vi "Main.vi"(8 "error in (no error)":errorcluster) -> (0 "error out":errorcluster)   [LabVIEW 2020, in "main.lvlib"]
uses:
  main.lvlib
  report format.ctl
  Module Data--cluster.ctl
  core/core_data/completed_tour.ctl
  core/core_data/chessboard_index.ctl
  core/core_data/tour type (enum).ctl
  core/core_data/chess_square--chess notation.ctl
  core/core_data/file--enum.ctl
  core/core_data/rank--enum.ctl
  config_buttons--enum.ctl
  update_completed_tour_text_indicator arguments.ctl
  create completed tour report (minimal).vi
  create completed tour report (detailed).vi
  <vilib>/Utility/error.llb/Clear Errors.vi
  core/core_wait (global variable).vi
  core/pause after every move (global variable).vi
  core/pause (global variable).vi
  convert--tour to string (minimal format).vi
  convert--tour to string (chessboard format).vi
  PTRL/string/Number (DBL) to comma delimited string.vi
  PTRL/dev_and_debug_tools/dev_and_debug_tools.lvlib
  PTRL/errors/errors.lvlib
  PTRL/GUI_tools/GUI_tools.lvlib
  queues/queue_core_loop/queue_core_loop.lvlib
  queues/queue_display_loop_1/queue_display_loop_1.lvlib
  global_stop_flag/global_stop_flag.lvlib
  app_data/app_data.lvlib
  status_text_indicator/Status_Text_Indicator.lvlib
  core/core.lvlib
  core/core_data/core_data.lvlib
  PTRL/timing_utilities/timing_utilities.lvlib
  app_log/app_log.lvlib
  PTRL/pro_dev_tools/pro_dev_tools.lvlib
  PTRL/string/string.lvlib
  stopwatch_timer/stopwatch_timer.lvlib
panel:
  out "avg. tour finding speed":string
  out "no. of completed tours":u64
  in  "Report format":T1
  in  "Log reports to file?":bool=TRUE caption="Log completed tour reports to file?"
  in  "open log in Sublime Text":bool
  in  "open log in Notepad":bool
  in  "open log folder":bool
  out "log file path":string caption="Log file path"
  out "avg. move speed":string
  out "no. of moves forward and backward in the last second":string
  out "total no. of moves":string
  out "total no. of moves backward":string
  out "total no. of moves forward":string
  in  "pause after every move?":bool caption="Pause after every move"
  in  "no. of ms to wait after each move":u32 max=5000 format="%d ms"
  out "no. of complete tours":string caption="no. of completed tours"
  out "complete_tour currently displayed":u64 caption="completed_tour currently displayed"
  in  "display_latest":bool=TRUE caption="Always show the latest completed tour"
  in  "display_previous":bool
  in  "display_next":bool
  out "complete_tour":string caption="Completed tour reports"
  out "running time":string
  out "total no. of moves":u64
  out "chessboard":bool[][](array[boolean]) caption="Chessboard"
  out "display loop 2":i32
  out "The tour":string caption="The current knight's tour"
  in  "Status":string
  in  "stop":bool
  in  "pause":bool
  in  "start":bool
  out "display loop 1":i32
  out "core loop":i32
  out "error case":errorcluster
  in  "top_left":u32(colorbox)=13434847
  in  "bottom_right":u32(colorbox)=16764108
  out "No. of states":i32
  out "MHL state transition (index 0 = oldest)":string[](array[string])
  out "MHL iteration":i32
  out "EHL iteration":i32
  out "Pre-loop init":errorcluster
  in  "Insert Unrecognised MHL command":bool
  in  "Insert error EHL":bool
  in  "Insert error MHL":bool
  # "Visible to user"
  # "Knight Tour"
  # "Tutorial section"
  # "Use the controls below to slow down the execution and/or to pause after every knight move."
  # "Invisible to user"
  # "8"
  # "7"
  # "6"
  # "5"
  # "4"
  # "3"
  # "2"
  # "1"
  # "a"
  # "b"
  # "c"
  # "d"
  # "e"
  # "f"
  # "g"
  # "h"
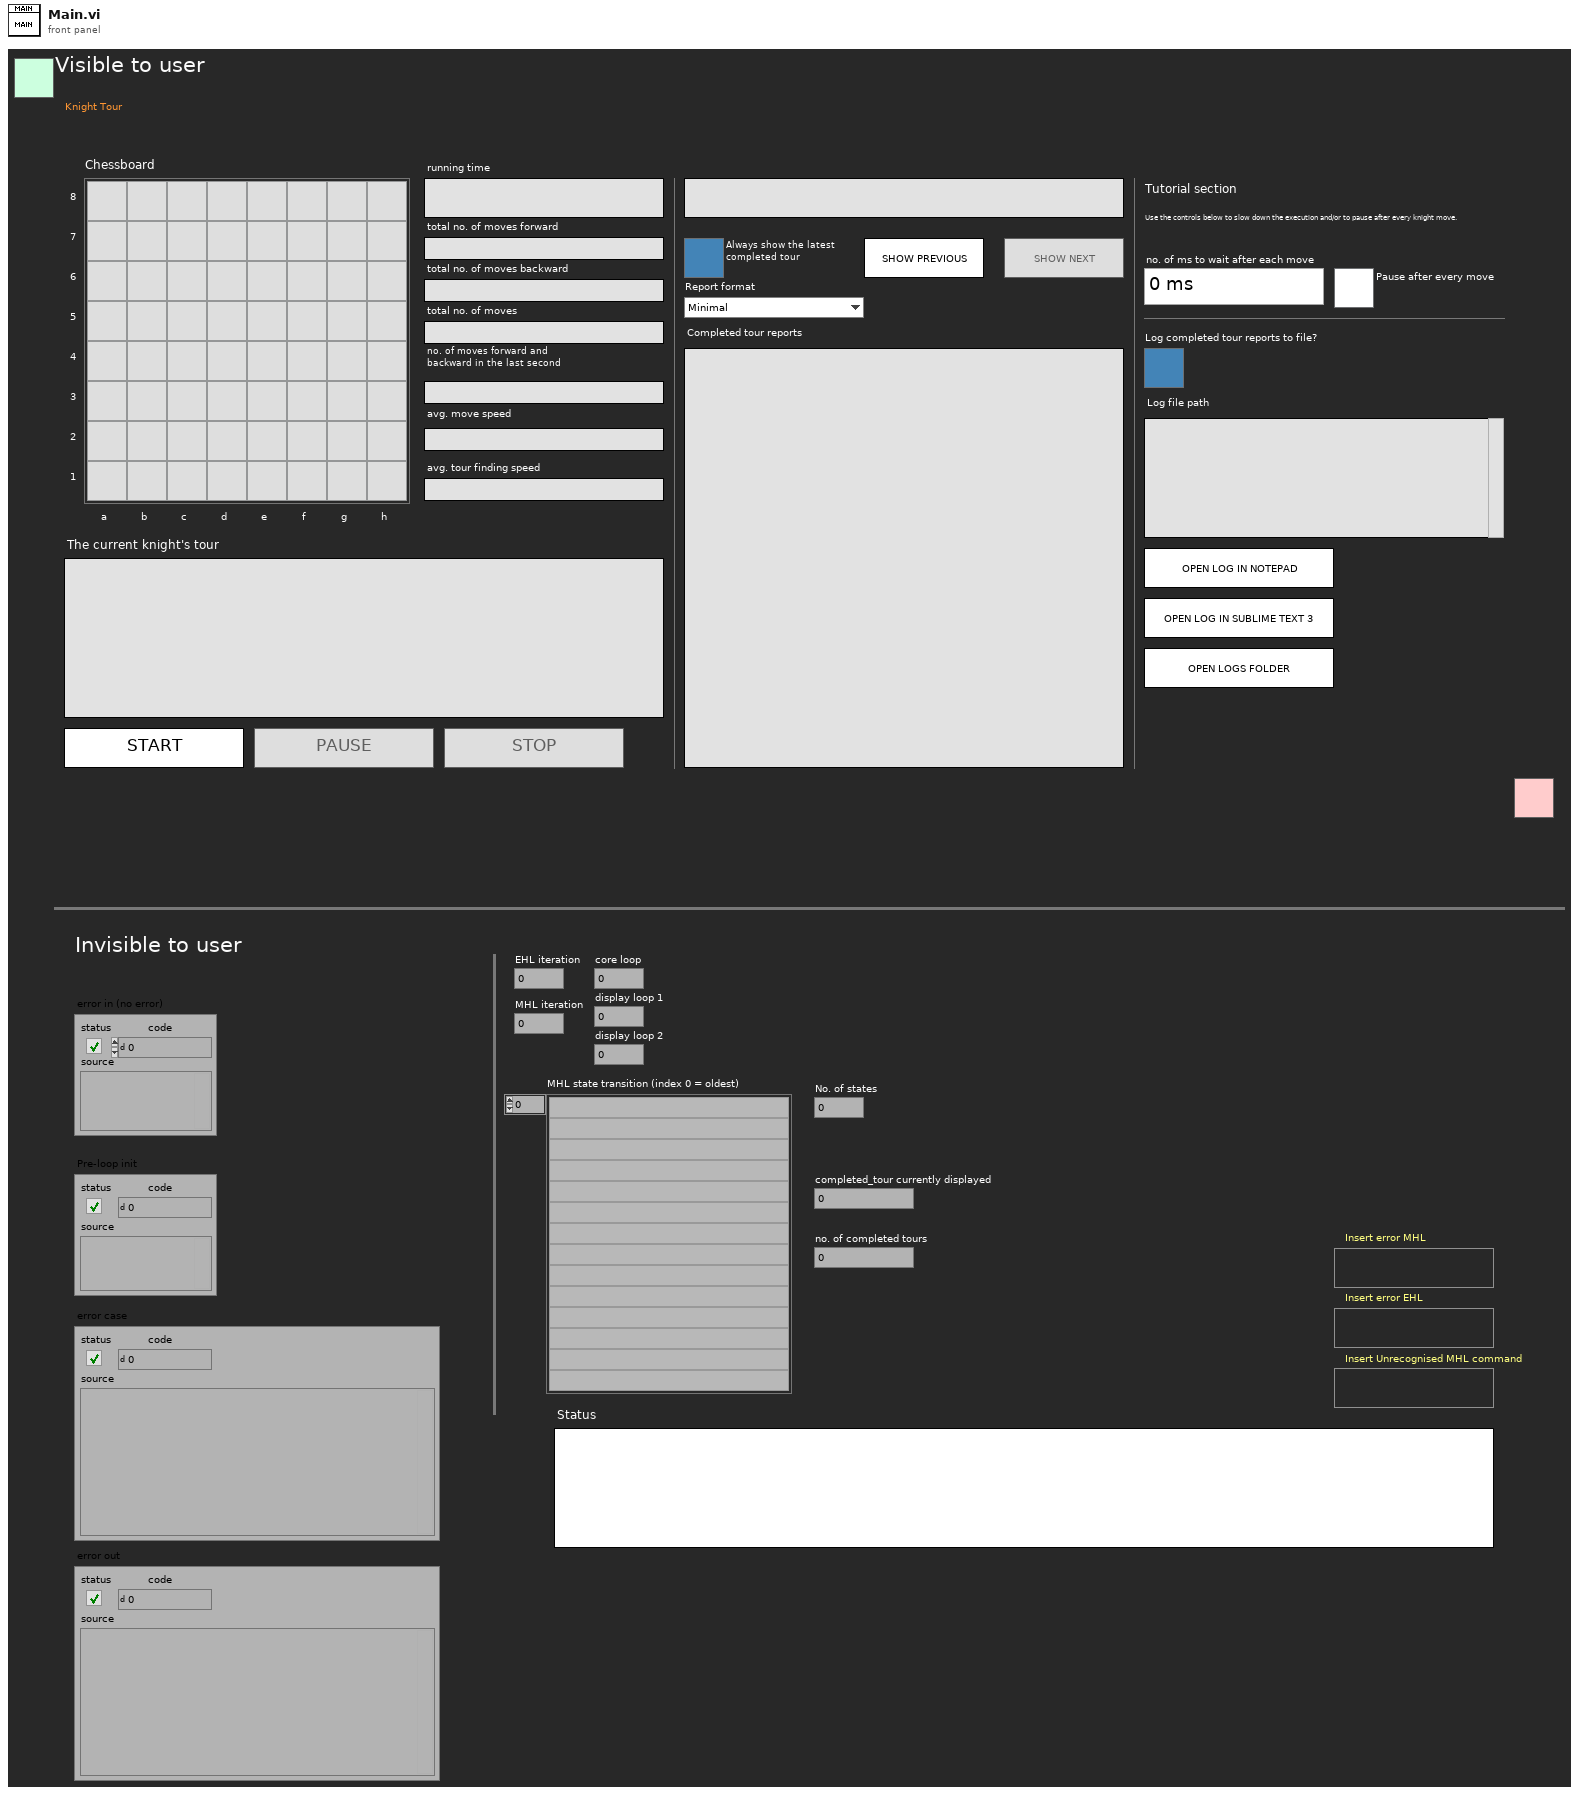
[diagram p1: front panel]
types:
  T1 = typedef "main.lvlib/report format.ctl" = enum16{"Minimal", "Detailed"}
  T2 = enum8{"Enabled", "Disabled", "Disabled and Grayed Out"}
  T3 = typedef "main.lvlib/Module Data--cluster.ctl" = cluster{"complete_tours":T4[], "no. of complete tours":u64, "complete_tour currently displayed":u64}
  T4 = typedef "core.lvlib/core_data.lvlib/completed_tour.ctl" = cluster{"complete_tour":T5[], "start square":string, "end square":string, "tour type":T6, "start_time":timestamp, "end_time":timestamp, "duration (seconds)":dbl, "duration (formatted string)":string, "no. of moves forward":u64, "no. of moves backward":u64, "total no. of moves since core started running":u64}
  T5 = typedef "core.lvlib/core_data.lvlib/chessboard_index.ctl" = cluster{"row":u8, "column":u8}
  T6 = typedef "core.lvlib/core_data.lvlib/tour type (enum).ctl" = enum16{"open", "closed"}
  T7 = typedef "main.lvlib/config_buttons--enum.ctl" = enum16{"tour_not_running", "tour_running", "tour_paused"}
  T8 = typedef "main.lvlib/update_completed_tour_text_indicator arguments.ctl" = cluster{"Completed tour paragraph":string, "tour number":u64}
  T9 = typedef "core.lvlib/core_data.lvlib/chess_square--chess notation.ctl" = cluster{"file":T10, "rank":T11}
  T10 = typedef "core.lvlib/core_data.lvlib/file--enum.ctl" = enum16{"a", "b", "c", "d", "e", "f", "g", "h"}
  T11 = typedef "core.lvlib/core_data.lvlib/rank--enum.ctl" = enum16{"1", "2", "3", "4", "5", "6", "7", "8"}
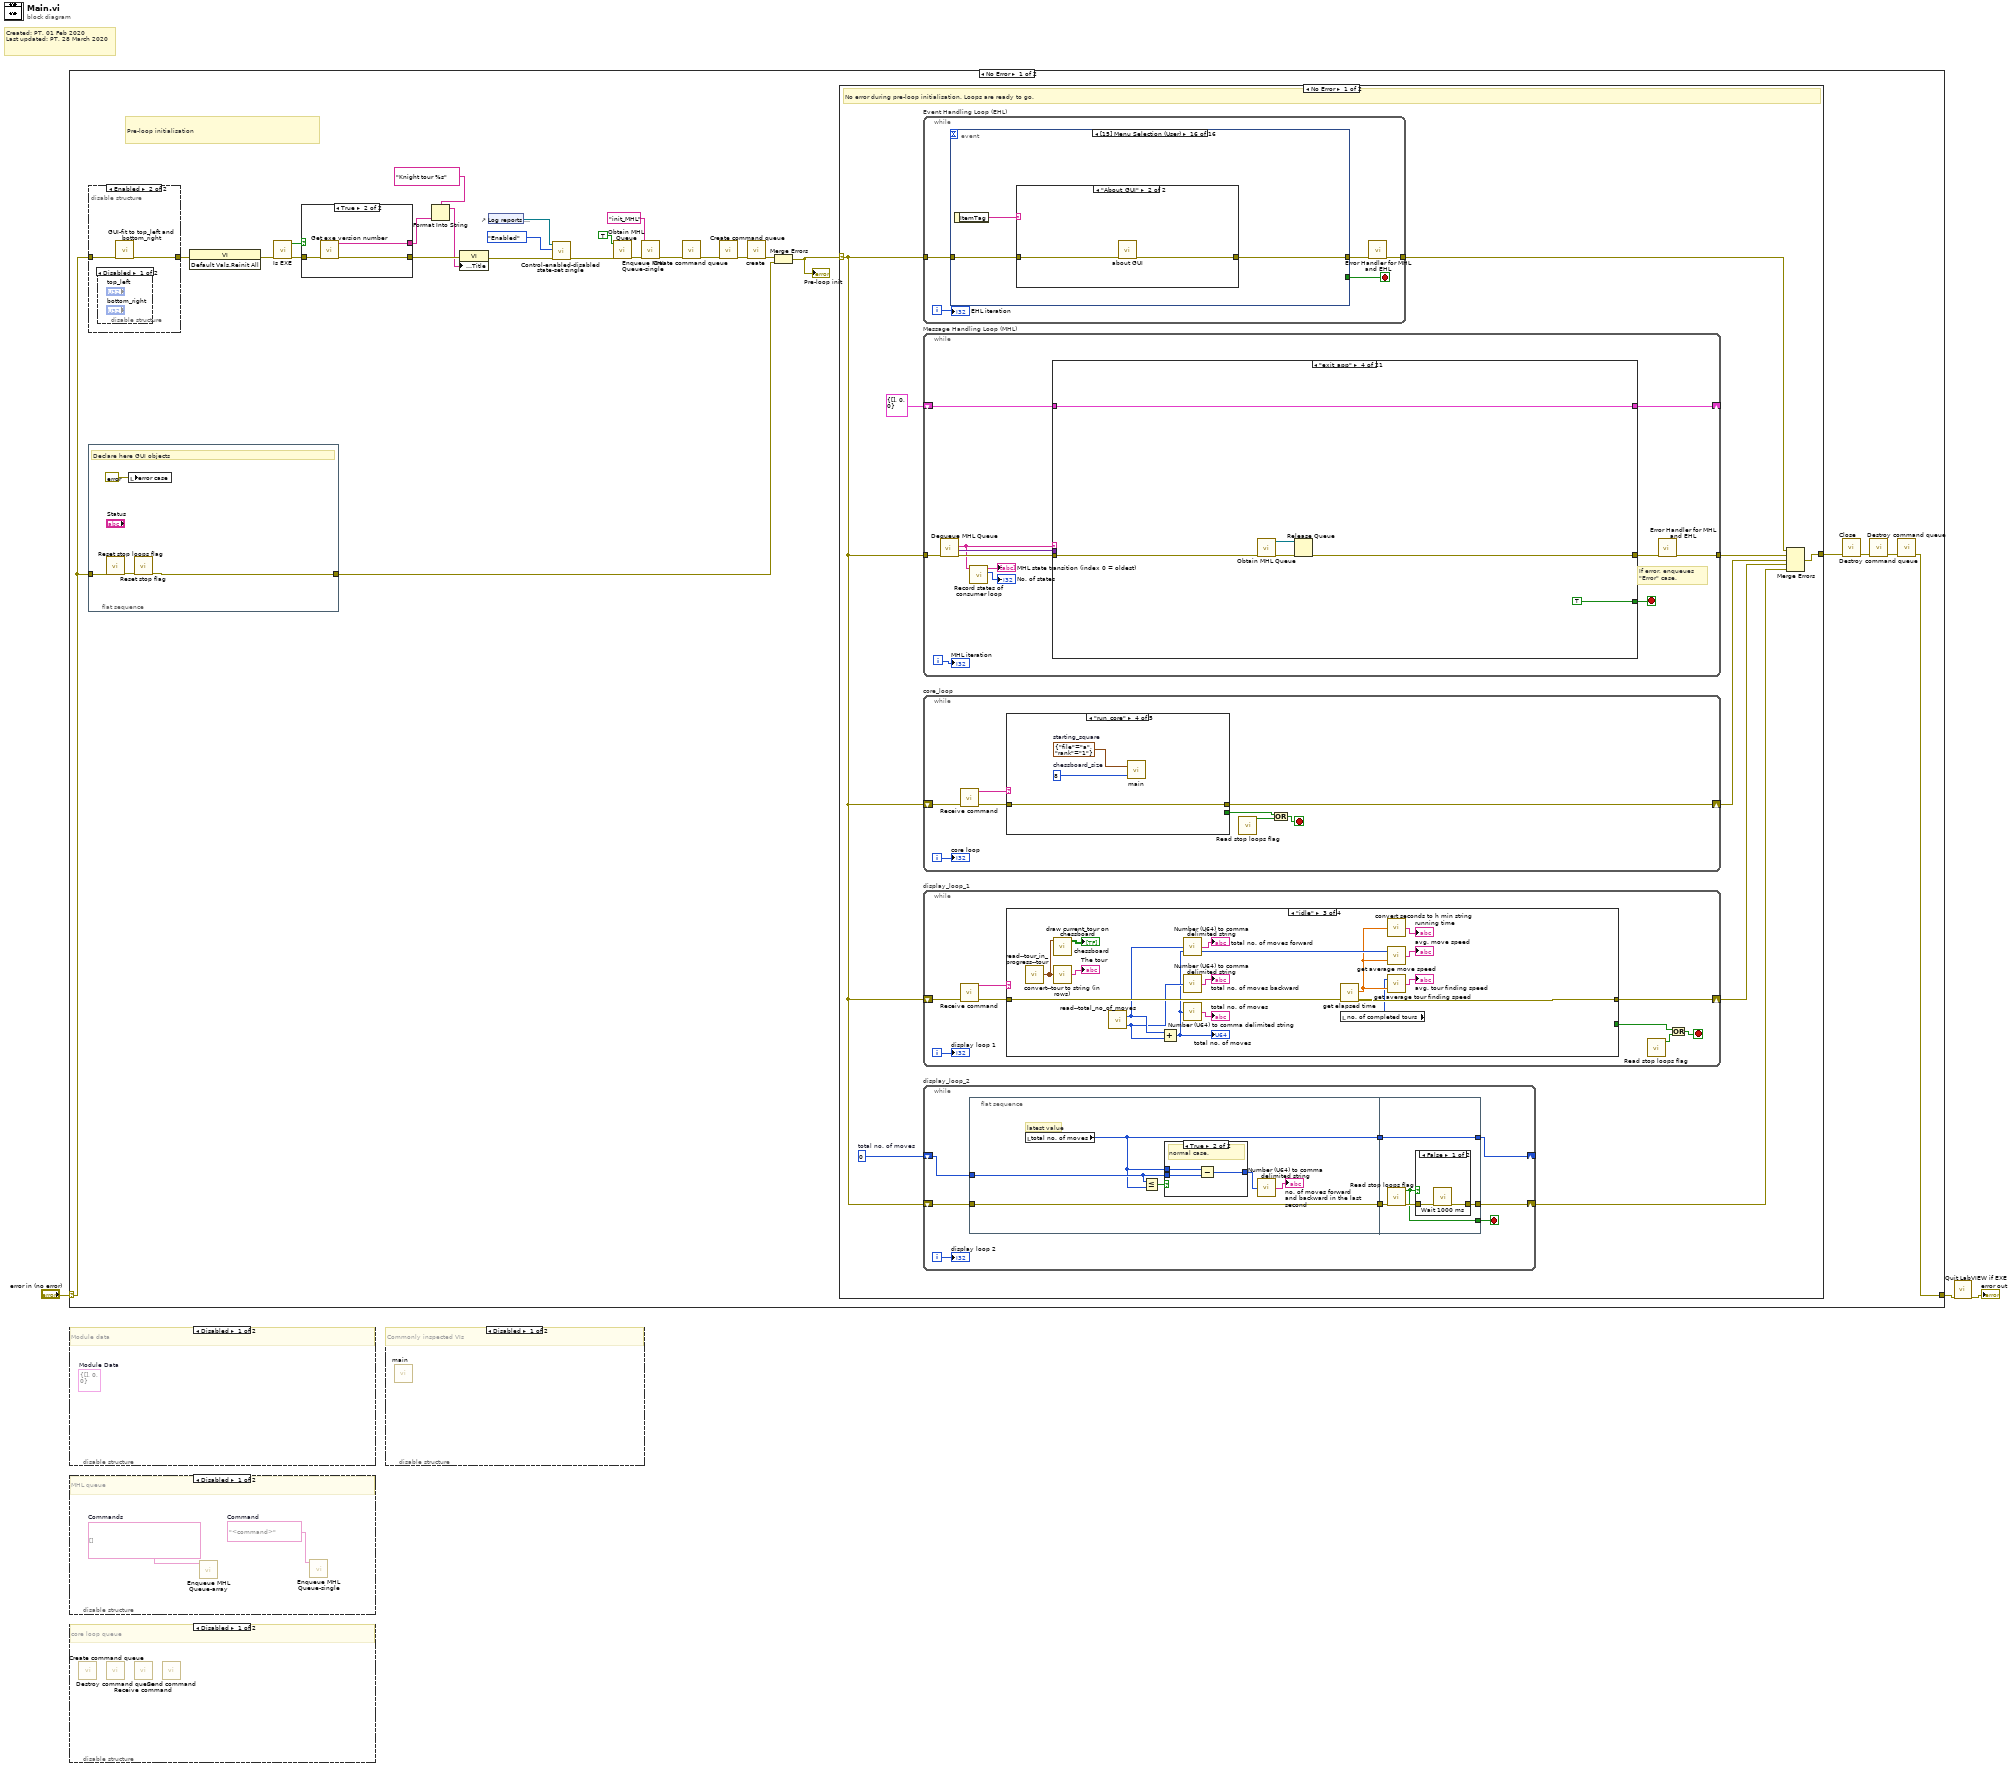
[diagram p0: block diagram]
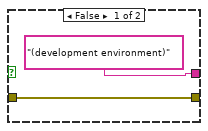
[diagram p2: hidden frame]
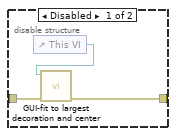
[diagram p3: hidden frame]
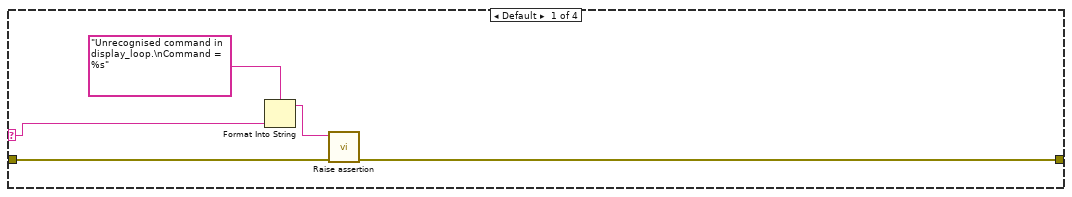
[diagram p5: hidden frame]
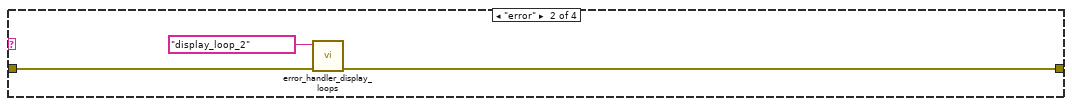
[diagram p6: hidden frame]
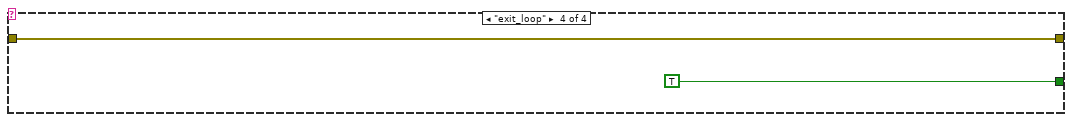
[diagram p7: hidden frame]
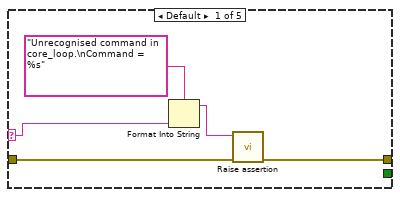
[diagram p8: hidden frame]
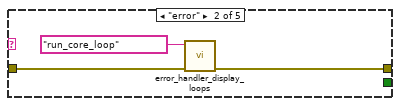
[diagram p9: hidden frame]
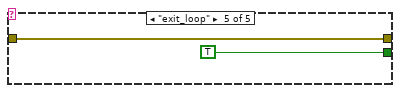
[diagram p11: hidden frame]
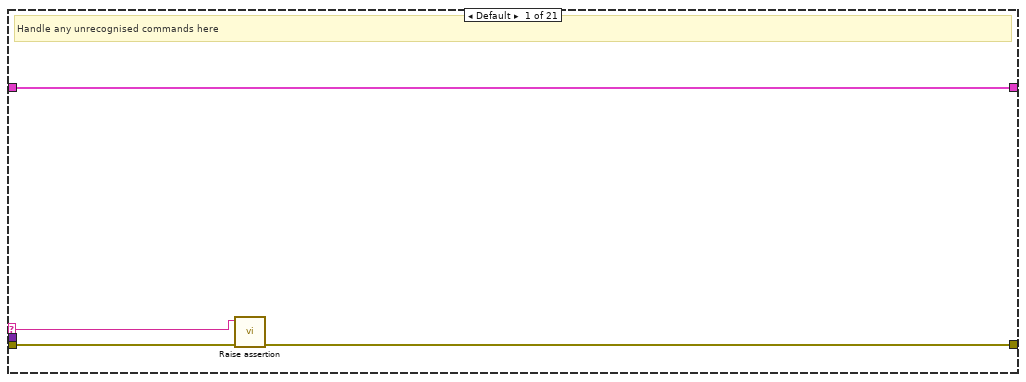
[diagram p12: hidden frame]
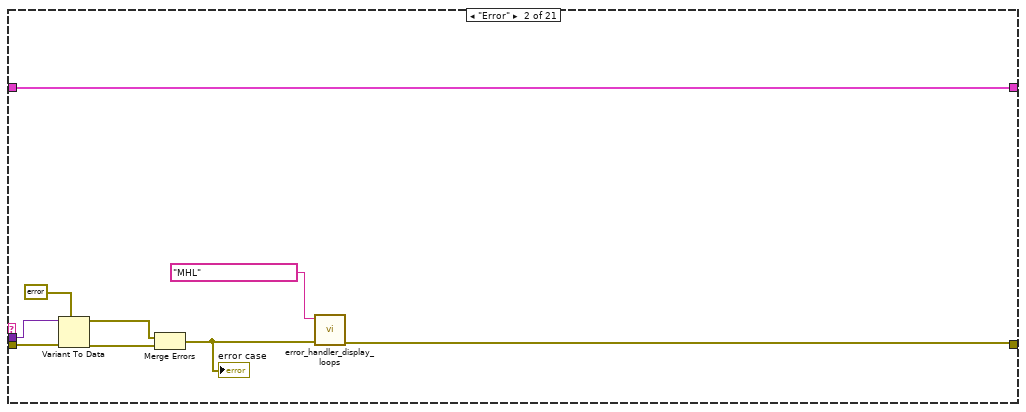
[diagram p13: hidden frame]
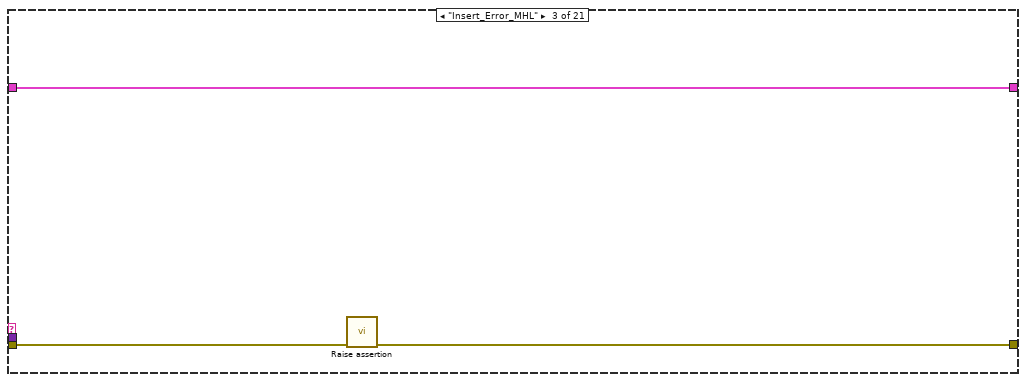
[diagram p14: hidden frame]
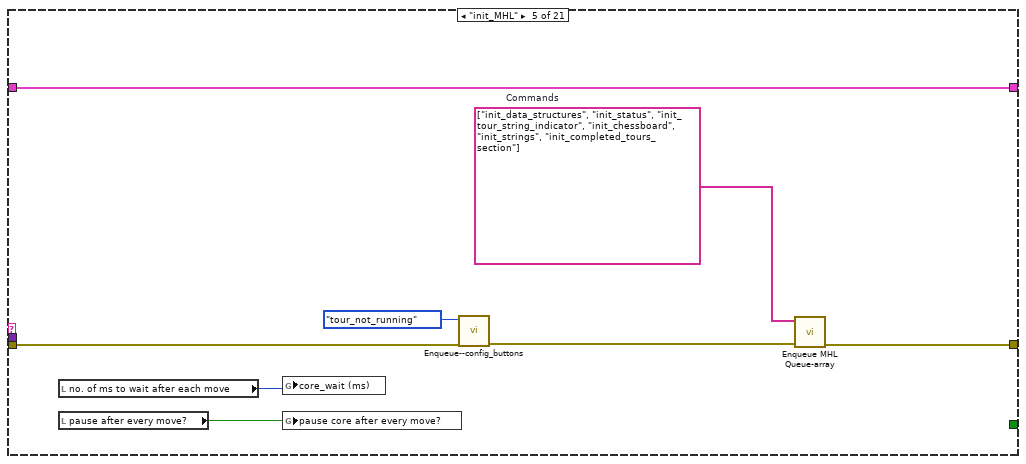
[diagram p15: hidden frame]
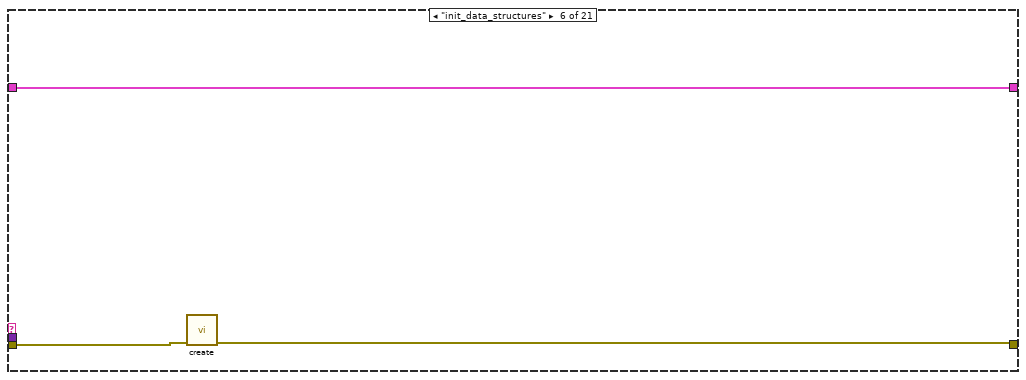
[diagram p16: hidden frame]
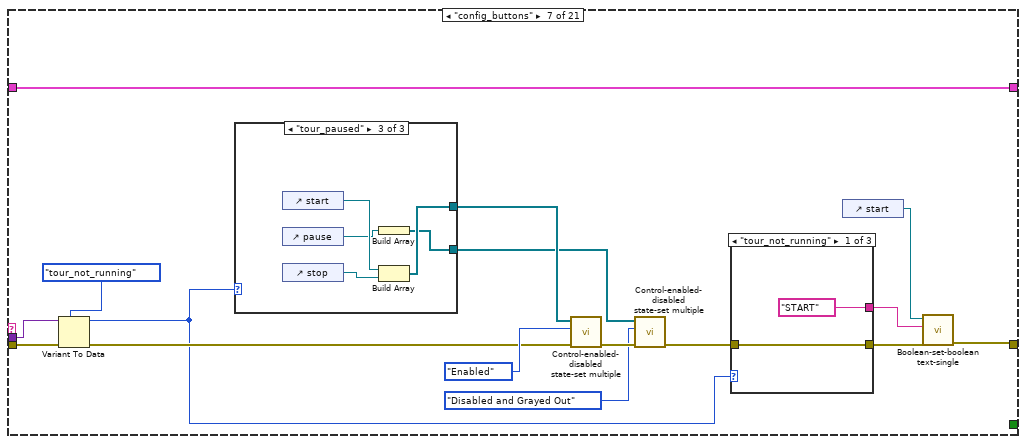
[diagram p17: hidden frame]
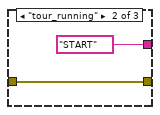
[diagram p18: hidden frame]
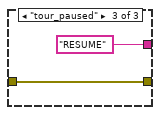
[diagram p19: hidden frame]
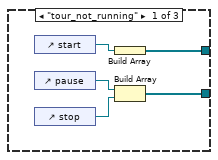
[diagram p20: hidden frame]
diagram:
  # "Created: PT, 01 Feb 2020\nLast updated: PT, 28 March 2020"
  n1 = case shown="No Error" "error in (no error)" {
    selector: "error in (no error)" -> [w24 w530]
    tunnel: [w29 w530] -> w2
    frame No Error {
      # "Pre-loop initialisation"
      n2 = disable-structure shown="Enabled" {
        disable-tunnel: w24 -> [w41 w43]
        disable-tunnel: [w40 w42] -> w27
        frame Disabled {
          n3 = control-ref of="This VI"() -> (w39:refnum<vi>)
          n4 = call "GUI-fit to largest decoration and center.vi"("error in (no error)"=w41, "VI Ref (calling VI)"=w39) -> ("error out"=w40:errorcluster)  [unwired: 9 in]
        }
        frame Enabled {
          n5 = disable-structure shown="Disabled" {
            frame Disabled {
            }
            frame Enabled {
            }
          }
          n6 = call "GUI-fit to top_left and bottom_right.vi"("error in (no error)"=w43) -> ("error out"=w42:errorcluster)  [unwired: 10 in]
        }
      }
      n7 = flat-sequence {
        tunnel: w24 -> [w37]
        tunnel: [w35] -> w22
        frame #0 {
          # "Declare here GUI objects"
          n8 = call "Reset stop loops flag.vi"("error in (no error)"=w37) -> ("error out"=w36:errorcluster)  [unwired: 10 in]
          n9 = local write "error case"(errorcluster {"status"=FALSE, "code"=0, "source"=""} ("error case")) -> ()
          n10 = call "Reset stop flag.vi"("error in (no error)"=w36) -> ("error out"=w35:errorcluster)  [unwired: 10 in]
        }
      }
      n11 = invoke class="VI" method="Default Vals.Reinit All"(error in=w27) -> (error out=w17:errorcluster)  [unwired: 2 in, 2 out]
      n12 = call "Is EXE.vi"("error in (no error)"=w17) -> ("error out"=w15:errorcluster, "T = is EXE"=w13:bool)  [unwired: 8 in, 1 out]
      n13 = case shown="True" w13 {
        tunnel: w15 -> [w31 w34]
        tunnel: [w31 w33] -> w14
        tunnel: ["(development environment)" w32] -> w10
        frame False {
        }
        frame True {
          n14 = call "Get exe version number.vi"("error in"=w34) -> ("error out"=w33:errorcluster, "EXE version number"=w32:string)  [unwired: 9 in]
        }
      }
      n15 = Format Into String(format string="Knight tour %s", w10) -> (resulting string=w11:string)  [unwired: 2 in, 1 out]
      n16 = property class="VI"(error in=w14, "Front Panel Window:Title"=w11) -> (error out=w16:errorcluster)  [unwired: 1 in, 1 out]
      n17 = control-ref of="Log reports to file?"() -> (w8:refnum<vi>)
      n18 = call "Control-enabled-disabled state-set single.vi"("error in (no error)"=w16, "State"=T2."Enabled", "Control ref in"=w8) -> ("error out"=w9:errorcluster)  [unwired: 7 in, 1 out]
      n19 = call "Obtain MHL Queue.vi"("ErrorIn"=w9, "Create New (F)"=TRUE) -> ("ErrorOut"=w28:errorcluster)  [unwired: 8 in, 1 out]
      n20 = call "Enqueue MHL Queue-single.vi"("ErrorIn"=w28, "Command"="init_MHL") -> ("ErrorOut"=w18:errorcluster)  [unwired: 9 in]
      n21 = call "Create command queue.vi"("error in (no error)"=w18) -> ("error out"=w21:errorcluster)  [unwired: 10 in]
      n22 = call "Create command queue.vi"("error in (no error)"=w21) -> ("error out"=w19:errorcluster)  [unwired: 10 in]
      n23 = call "create.vi"("error in"=w19) -> ("error out"=w6:errorcluster)  [unwired: 10 in]
      n24 = Merge Errors(w6, w22) -> (w23:errorcluster)
      "Pre-loop init" <- w23
      n25 = case shown="No Error" w23 {
        selector: w23 -> [w44 w529]
        tunnel: [w51 w529] -> w5
        frame No Error {
          w45 = u64 0  # total no. of moves
          # "No error during pre-loop initialisation. Loops are ready to go."
          n26 = while "Event Handling Loop (EHL)" {
            tunnel: w44 -> [w404]
            tunnel: [w402] -> w52
            i -> [w400]
            stop <- w403 stop-if-true
            n27 = event shown="[15] Menu Selection (User)" {
              selector: _ -> [_ _ _ _ _ _ _ _ _ _ _ _ _ _ _ _]
              dyn-events: _ -> [_ _ _ _ _ _ _ _ _ _ _ _ _ _ _ _]
              timeout: _ -> [_ _ _ _ _ _ _ _ _ _ _ _ _ _ _ _]
              tunnel: w404 -> [w407 w420 w422 w425 w428 w434 w437 w444 w451 w454 w456 w458 w462 w474 w487 w500]
              tunnel: [w405 _ _ _ _ _ _ _ _ _ _ _ _ _ _ _] -> w403
              tunnel: [w409 w421 w423 w426 w432 w435 w441 w443 w450 w453 w456 w458 w463 w473 w486 w499] -> w401
              event Panel Close? {
                n28 = event-data() -> ()  [unwired: 1 in, 1 out]
                n29 = call "dialogue--exit_app.vi"("error in (no error)"=w407) -> ("error out"=w408:errorcluster, "T = exit was pressed"=w406:bool)  [unwired: 9 in]
                n30 = case shown="True" w406 {
                  tunnel: w408 -> [w411 w418]
                  tunnel: [w411 w416] -> w409
                  tunnel: [_ TRUE] -> w405
                  frame False {
                  }
                  frame True {
                    w413 = "exit_loop" ("command")
                    n31 = call "Enqueue--exit_app.vi"("error in (no error)"=w418) -> ("error out"=w415:errorcluster)  [unwired: 10 in]
                    n32 = call "Send command.vi"("error in (no error)"=w415, "command"=w413) -> ("error out"=w414:errorcluster)  [unwired: 9 in]
                    n33 = call "Send command.vi"("error in (no error)"=w414, "command"=w413) -> ("error out"=w412:errorcluster)  [unwired: 9 in]
                    n34 = call "Set stop loops flag.vi"("error in (no error)"=w412) -> ("error out"=w416:errorcluster)  [unwired: 10 in]
                  }
                }
                n35 = event-data("Discard?"=TRUE) -> ()  [unwired: 1 in, 1 out]
              }
              event "Insert error MHL": Value Change {
                # "This case is very useful to simulate the behaviour of the MHL (and of the GUI as a whole), when an error happens in the MHL loop."
                n36 = event-data() -> ()  [unwired: 1 in, 1 out]
                n37 = call "Enqueue MHL Queue-single.vi"("ErrorIn"=w420, "Command"="Insert_Error_MHL") -> ("ErrorOut"=w421:errorcluster)  [unwired: 9 in]
              }
              event "Insert error EHL": Value Change {
                # "This case is very useful to simulate the behaviour of the EHL (and of the GUI as a whole), when an error happens in the EHL loop."
                n38 = event-data() -> ()  [unwired: 1 in, 1 out]
                n39 = call "Raise assertion.vi"("error in (no error)"=w422) -> ("error out"=w423:errorcluster)  [unwired: 10 in]
              }
              event "Insert Unrecognised MHL command": Value Change {
                w424 = "abcd1234xyzw"  # Command
                # "This case is very useful to simulate the behaviour of the MHL (and of the GUI as a whole), when an unrecognised message is enqueued to the MHL loop."
                n40 = event-data() -> ()  [unwired: 1 in, 1 out]
                n41 = call "Enqueue MHL Queue-single.vi"("ErrorIn"=w425, "Command"=w424) -> ("ErrorOut"=w426:errorcluster)  [unwired: 9 in]
              }
              event "start": Value Change {
                # "Disable such that user cannot change the \"log to file?\" option while the core is running. The user can change it when the app first starts (before START is pressed) or when the core is stopped."
                n42 = event-data() -> ()  [unwired: 1 in, 1 out]
                n43 = control-ref of="Log reports to file?"() -> (w429:refnum<vi>)
                n44 = call "Control-enabled-disabled state-set single.vi"("error in (no error)"=w428, "State"=T2."Disabled and Grayed Out", "Control ref in"=w429) -> ("error out"=w427:errorcluster)  [unwired: 7 in, 1 out]
                n45 = call "Enqueue MHL Queue-single.vi"("ErrorIn"=w427, "Command"="button_press_start") -> ("ErrorOut"=w432:errorcluster)  [unwired: 9 in]
              }
              event "pause": Value Change {
                n46 = event-data() -> ()  [unwired: 1 in, 1 out]
                n47 = call "Enqueue MHL Queue-single.vi"("ErrorIn"=w434, "Command"="button_press_pause") -> ("ErrorOut"=w435:errorcluster)  [unwired: 9 in]
              }
              event "stop": Value Change {
                # "Re-enable the button, enabling the user would to chance the \"log to file?\" option before the user restarts the core."
                n48 = event-data() -> ()  [unwired: 1 in, 1 out]
                n49 = control-ref of="Log reports to file?"() -> (w438:refnum<vi>)
                n50 = call "Control-enabled-disabled state-set single.vi"("error in (no error)"=w437, "State"=T2."Enabled", "Control ref in"=w438) -> ("error out"=w436:errorcluster)  [unwired: 7 in, 1 out]
                n51 = call "Enqueue MHL Queue-single.vi"("ErrorIn"=w436, "Command"="button_press_stop") -> ("ErrorOut"=w441:errorcluster)  [unwired: 9 in]
              }
              event "display_latest": Value Change {
                n52 = event-data() -> ("NewVal"=w442:bool)  [unwired: 1 in]
                n53 = case shown="True" w442 {
                  tunnel: w444 -> [w445 w448]
                  tunnel: [w445 w447] -> w443
                  frame False {
                  }
                  frame True {
                    n54 = call "Enqueue MHL Queue-single.vi"("ErrorIn"=w448, "Command"="display_latest_completed_tour") -> ("ErrorOut"=w447:errorcluster)  [unwired: 9 in]
                  }
                }
              }
              event "display_next": Value Change {
                n55 = event-data() -> ()  [unwired: 1 in, 1 out]
                n56 = call "Enqueue MHL Queue-single.vi"("ErrorIn"=w451, "Command"="display_next_button_press") -> ("ErrorOut"=w450:errorcluster)  [unwired: 9 in]
              }
              event "display_previous": Value Change {
                n57 = event-data() -> ()  [unwired: 1 in, 1 out]
                n58 = call "Enqueue MHL Queue-single.vi"("ErrorIn"=w454, "Command"="display_previous_button_press") -> ("ErrorOut"=w453:errorcluster)  [unwired: 9 in]
              }
              event "no. of ms to wait after each move": Value Change {
                n59 = event-data() -> ("NewVal"=w455:u32)  [unwired: 1 in]
                n60 = global write "core_wait (global variable).vi" "core_wait (ms)"(w455) -> ()
              }
              event "pause after every move?": Value Change {
                n61 = event-data() -> ("NewVal"=w457:bool)  [unwired: 1 in]
                n62 = global write "pause after every move (global variable).vi" "pause core after every move?"(w457) -> ()
              }
              event "open log folder": Value Change {
                n63 = event-data() -> ()  [unwired: 1 in, 1 out]
                n64 = local read "log file path"() -> (w461:string)
                n65 = Empty String/Path?(string/path=w461) -> (empty?=w460:bool)
                n66 = Not(x=w460) -> (.not. x?=w459:bool)
                n67 = case shown="False" w459 {
                  tunnel: [w465 w469] -> w463
                  tunnel: w462 -> [w464 w468]
                  tunnel: w461 -> [_ w467]
                  frame False {
                    n68 = call "dialogue--there is no log file.vi"("error in (no error)"=w464) -> ("error out"=w465:errorcluster)  [unwired: 10 in]
                  }
                  frame True {
                    n69 = String To Path(string=w467) -> (path=w466:path)
                    n70 = call <vilib>:"Show in File System.vi"("error in (no error)"=w468, "file or directory path"=w466) -> ("error out"=w469:errorcluster)  [unwired: 9 in]
                  }
                }
              }
              event "open log in Notepad": Value Change {
                n71 = event-data() -> ()  [unwired: 1 in, 1 out]
                n72 = local read "log file path"() -> (w472:string)
                n73 = Empty String/Path?(string/path=w472) -> (empty?=w471:bool)
                n74 = Not(x=w471) -> (.not. x?=w470:bool)
                n75 = case shown="True" w470 {
                  tunnel: w474 -> [w476 w480]
                  tunnel: [w475 w479] -> w473
                  tunnel: w472 -> [_ w478]
                  frame False {
                    n76 = call "dialogue--there is no log file.vi"("error in (no error)"=w476) -> ("error out"=w475:errorcluster)  [unwired: 10 in]
                  }
                  frame True {
                    n77 = Format Into String(format string="notepad.exe \"%s\"", w478) -> (resulting string=w481:string)  [unwired: 2 in, 1 out]
                    n78 = call <vilib>:"System Exec.vi"("wait until completion? (T)"=FALSE, "error in (no error)"=w480, "command line"=w481) -> ("error out"=w479:errorcluster)  [unwired: 5 in, 3 out]
                  }
                }
              }
              event "open log in Sublime Text": Value Change {
                n79 = event-data() -> ()  [unwired: 1 in, 1 out]
                n80 = local read "log file path"() -> (w485:string)
                n81 = Empty String/Path?(string/path=w485) -> (empty?=w484:bool)
                n82 = Not(x=w484) -> (.not. x?=w483:bool)
                n83 = case shown="False" w483 {
                  tunnel: w487 -> [w489 w496]
                  tunnel: [w488 w495] -> w486
                  tunnel: w485 -> [_ w491]
                  frame False {
                    n84 = call "dialogue--there is no log file.vi"("error in (no error)"=w489) -> ("error out"=w488:errorcluster)  [unwired: 10 in]
                  }
                  frame True {
                    w490 = "\""
                    w494 = "C:\\Program Files\\Sublime Text 3\\subl.exe"  # The Sublime Text installation folder is assumed to be "C:\Program Files\Sublime Text 3" and is hardcoded. Not an ideal implementation, but should work for the majority of people that use Sublime Text 3.
                    n85 = call <vilib>:"Space Constant.vi"() -> ("String"=w493:string)
                    n86 = Concatenate Strings(w494, w493, w490, w491, w490) -> (w492:string)
                    n87 = call <vilib>:"System Exec.vi"("wait until completion? (T)"=FALSE, "error in (no error)"=w496, "command line"=w492) -> ("error out"=w495:errorcluster)  [unwired: 5 in, 3 out]
                  }
                }
              }
              event Menu Selection (User) {
                n88 = event-data() -> ("ItemTag"=w498:string)  [unwired: 1 in]
                n89 = case shown="\"About_GUI\"" w498 {
                  tunnel: w500 -> [w501 w503]
                  tunnel: [w501 w502] -> w499
                  frame Default {
                  }
                  frame "About_GUI" {
                    n90 = call "about GUI.vi"("error in (no error)"=w503) -> ("error out"=w502:errorcluster)  [unwired: 10 in]
                  }
                }
              }
            }
            n91 = call "Error Handler for MHL and EHL.vi"("ErrorIn"=w401) -> ("ErrorOut"=w402:errorcluster)  [unwired: 10 in]
            "EHL iteration" <- w400
          }
          n92 = while "Message Handling Loop (MHL)" {
            tunnel: [w117] -> w47
            tunnel: w44 -> [w116]
            shift-right: [w110] -> _
            shift-left: T3 {"complete_tours"=[], "no. of complete tours"=0, "complete_tour currently displayed"=0} ("Module Data") -> [w109]
            i -> [w114]
            stop <- w120 stop-if-true
            # "If error, enqueues \"Error\" case."
            n93 = call "Dequeue MHL Queue.vi"("ErrorIn"=w116) -> ("ErrorOut"=w118:errorcluster, "Data"=w115:variant, "Command"=w113:string)  [unwired: 8 in]
            n94 = call "Record states of consumer loop.vi"("State in"=w113) -> ("No. of states"=→"No. of states":i32, "States out (index 0 = oldest)"=→"MHL state transition (index 0 = oldest)":string[])  [unwired: 8 in, 1 out]
            n95 = case shown="\"exit_app\"" w113 {
              selector: w113 -> [w122 _ _ _ _ _ _ _ _ _ _ _ _ _ _ _ _ _ _ _ _]
              tunnel: w118 -> [w124 w133 w135 w140 w146 w151 w169 w194 w203 w206 w216 w234 w245 w282 w290 w312 w334 w355 w368 w373 w388]
              tunnel: [w123 w126 w136 w141 w149 w152 w157 w191 w198 w206 w213 w227 w249 w285 w288 w309 w329 w352 w361 w372 w387] -> w119
              tunnel: [_ _ _ TRUE _ _ _ _ _ _ _ _ _ _ _ _ _ _ _ _ _] -> w120
              tunnel: w115 -> [_ w131 _ _ _ _ w163 _ _ _ _ _ _ _ _ w311 _ w350 w367 _ _]
              tunnel: [w121 w129 w134 w137 w150 w153 w168 w195 w202 w205 w217 w233 w242 w287 w294 w306 w333 w354 w363 w374 w389] -> w110
              tunnel: w109 -> [w121 w129 w134 w137 w150 w153 w168 w195 w202 w205 w217 w233 w243 w287 w294 w305 w333 w354 w358 w374 w389]
              frame Default {
                # "Handle any unrecognised commands here"
                n96 = call "Raise assertion.vi"("error in (no error)"=w124, "Details (dflt=\"no details\")"=w122) -> ("error out"=w123:errorcluster)  [unwired: 9 in]
              }
              frame "Error" {
                n97 = Variant To Data(error in=w133, type=errorcluster {"status"=FALSE, "code"=0, "source"=""} ("error constant"), Variant=w131) -> (data=w128:errorcluster, error out=w130:errorcluster)
                n98 = Merge Errors(w128, w130) -> (w127:errorcluster)
                "error case" <- w127
                n99 = call "error_handler_display_loops.vi"("error in (no error)"=w127, "Name of VI or Module"="MHL") -> ("error out"=w126:errorcluster)  [unwired: 9 in]
              }
              frame "Insert_Error_MHL" {
                n100 = call "Raise assertion.vi"("error in (no error)"=w135) -> ("error out"=w136:errorcluster)  [unwired: 10 in]
              }
              frame "exit_app" {
                n101 = call "Obtain MHL Queue.vi"("ErrorIn"=w140) -> ("ErrorOut"=w139:errorcluster, "MHL Queue Out"=w138:refnum<queue>)  [unwired: 9 in]
                n102 = Release Queue(queue=w138, error in (no error)=w139) -> (error out=w141:errorcluster)  [unwired: 1 in, 2 out]
              }
              frame "init_MHL" {
                w148 = string[] ["init_data_structures", "init_status", "init_tour_string_indicator", "init_chessboard", "init_strings", "init_completed_tours_section"]  # Commands
                n103 = local read "no. of ms to wait after each move"() -> (w144:u32)
                n104 = local read "pause after every move?"() -> (w143:bool)
                n105 = global write "core_wait (global variable).vi" "core_wait (ms)"(w144) -> ()
                n106 = global write "pause after every move (global variable).vi" "pause core after every move?"(w143) -> ()
                n107 = call "Enqueue--config_buttons.vi"("error in (no error)"=w146, "config_buttons"=config_buttons--enum."tour_not_running") -> ("error out"=w147:errorcluster)  [unwired: 9 in]
                n108 = call "Enqueue MHL Queue-array.vi"("error in (no error)"=w147, "Commands"=w148) -> ("error out"=w149:errorcluster)  [unwired: 9 in]
              }
              frame "init_data_structures" {
                n109 = call "create.vi"("error in (no error)"=w151) -> ("error out"=w152:errorcluster)  [unwired: 10 in]
              }
              frame "config_buttons" {
                n110 = Variant To Data(error in=w169, type=config_buttons--enum."tour_not_running" ("config_buttons"), Variant=w163) -> (data=w158:T7, error out=w164:errorcluster)
                n111 = case shown="\"tour_paused\"" w158 {
                  tunnel: [w179 w181 w188] -> w160
                  tunnel: [w176 w184 w186] -> w159
                  frame "tour_not_running" {
                    n112 = control-ref of="start"() -> (w180:refnum<vi>)
                    n113 = control-ref of="pause"() -> (w178:refnum<vi>)
                    n114 = control-ref of="stop"() -> (w177:refnum<vi>)
                    n115 = Build Array(w180) -> (w179:refnum<vi>[])
                    n116 = Build Array(w178, w177) -> (w176:refnum<vi>[])
                  }
                  frame "tour_running" {
                    n117 = control-ref of="start"() -> (w185:refnum<vi>)
                    n118 = control-ref of="pause"() -> (w183:refnum<vi>)
                    n119 = control-ref of="stop"() -> (w182:refnum<vi>)
                    n120 = Build Array(w185) -> (w184:refnum<vi>[])
                    n121 = Build Array(w183, w182) -> (w181:refnum<vi>[])
                  }
                  frame "tour_paused" {
                    n122 = control-ref of="start"() -> (w190:refnum<vi>)
                    n123 = control-ref of="pause"() -> (w187:refnum<vi>)
                    n124 = control-ref of="stop"() -> (w189:refnum<vi>)
                    n125 = Build Array(w187) -> (w186:refnum<vi>[])
                    n126 = Build Array(w190, w189) -> (w188:refnum<vi>[])
                  }
                }
                n127 = call "Control-enabled-disabled state-set multiple.vi"("error in (no error)"=w164, "State"=T2."Enabled", "Control refs in"=w160) -> ("error out"=w167:errorcluster)  [unwired: 7 in, 1 out]
                n128 = call "Control-enabled-disabled state-set multiple.vi"("error in (no error)"=w167, "State"=T2."Disabled and Grayed Out", "Control refs in"=w159) -> ("error out"=w166:errorcluster)  [unwired: 7 in, 1 out]
                n129 = case shown="\"tour_not_running\"" w158 {
                  tunnel: w166 -> [w171 w173 w175]
                  tunnel: [w171 w173 w175] -> w156
                  tunnel: ["START" "START" "RESUME"] -> w154
                  frame "tour_not_running" {
                  }
                  frame "tour_running" {
                  }
                  frame "tour_paused" {
                  }
                }
                n130 = control-ref of="start"() -> (w155:refnum<vi>)
                n131 = call "Boolean-set-boolean text-single.vi"("error in (no error)"=w156, "Boolean Text"=w154, "Boolean ref in"=w155) -> ("error out"=w157:errorcluster)  [unwired: 7 in, 1 out]
              }
              frame "init_status" {
                n132 = control-ref of="Status"() -> (w192:refnum<vi>)
                n133 = call "Init.vi"("error in (no error)"=w194, "Status_Text_Indicator"=w192) -> ("error out"=w193:errorcluster)  [unwired: 9 in]
                n134 = call "Clear status.vi"("error in (no error)"=w193) -> ("error out"=w191:errorcluster)  [unwired: 10 in]
              }
              frame "init_tour_string_indicator" {
                n135 = control-ref of="The tour"() -> (w200:refnum<vi>)
                n136 = call "String-set-font type.vi"("error in (no error)"=w203, "Font:Name"="Consolas", "String ref in"=w200) -> ("error out"=w201:errorcluster, "String ref out"=w197:refnum<vi>)  [unwired: 7 in]
                n137 = call "String-set-font size.vi"("error in (no error)"=w201, "Text.Font:Size (Dflt=15pt)"=u32 20, "String ref in"=w197) -> ("error out"=w198:errorcluster)  [unwired: 7 in, 1 out]
              }
              frame "init_chessboard" {
                w204 = bool[][] []  # empty array
                n138 = local write "chessboard"(w204) -> ()
              }
              frame "init_strings" {
                n139 = control-ref of="running time"() -> (w214:refnum<vi>)
                n140 = call "String-set font type and size-Consolas 30.vi"("error in (no error)"=w216, "String"=w214) -> ("error out"=w215:errorcluster)  [unwired: 9 in]
                n141 = control-ref of="total no. of moves forward"() -> (w212:refnum<vi>)
                n142 = control-ref of="total no. of moves backward"() -> (w211:refnum<vi>)
                n143 = control-ref of="total no. of moves"() -> (w210:refnum<vi>)
                n144 = control-ref of="no. of moves forward and backward in the last second"() -> (w209:refnum<vi>)
                n145 = control-ref of="avg. move speed"() -> (w208:refnum<vi>)
                n146 = Build Array(w212, w211, w210, w209, w208) -> (w207:refnum<vi>[])
                n147 = for {
                  shift-right: [w219] -> w213
                  shift-left: w215 -> [w220]
                  tunnel: w207 -> [w218] mode=indexing
                  n148 = call "String-set font type and size-Consolas 15.vi"("error in (no error)"=w220, "String"=w218) -> ("error out"=w219:errorcluster)  [unwired: 9 in]
                }
              }
              frame "init_completed_tours_section" {
                n149 = flat-sequence {
                  tunnel: w234 -> [w241]
                  tunnel: [w241] -> w232
                  frame #0 {
                    # "These GUI objects form the \"completed tours section\" of the GUI."
                    n150 = local write "display_latest"(TRUE ("display_latest")) -> ()
                    n151 = local write "complete_tour"("") -> ()
                    n152 = local write "no. of complete tours"("No tours found" ("no. of completed tours")) -> ()
                  }
                }
                n153 = control-ref of="display_next"() -> (w231:refnum<vi>)
                n154 = control-ref of="display_previous"() -> (w230:refnum<vi>)
                n155 = Build Array(w231, w230) -> (w229:refnum<vi>[])
                n156 = call "Control-enabled-disabled state-set multiple.vi"("error in (no error)"=w232, "State"=T2."Disabled and Grayed Out", "Control refs in"=w229) -> ("error out"=w224:errorcluster)  [unwired: 7 in, 1 out]
                n157 = control-ref of="no. of complete tours"() -> (w225:refnum<vi>)
                n158 = call "String-set font type and size-Consolas 30.vi"("error in (no error)"=w224, "String"=w225) -> ("error out"=w223:errorcluster)  [unwired: 9 in]
                n159 = control-ref of="complete_tour"() -> (w226:refnum<vi>)
                n160 = control-ref of="log file path"() -> (w221:refnum<vi>)
                n161 = Build Array(w226, w221) -> (w222:refnum<vi>[])
                n162 = for {
                  tunnel: w222 -> [w236] mode=indexing
                  shift-right: [w237] -> w227
                  shift-left: w223 -> [w235]
                  n163 = call "String-set font type and size-Consolas 15.vi"("error in (no error)"=w235, "String"=w236) -> ("error out"=w237:errorcluster)  [unwired: 9 in]
                }
              }
              frame "button_press_start" {
                n164 = flat-sequence {
                  tunnel: w245 -> [w252]
                  tunnel: [w251] -> w244
                  frame #0 {
                    n165 = call "Reset stop flag.vi"("error in (no error)"=w252) -> ("error out"=w251:errorcluster)  [unwired: 10 in]
                    n166 = global write "pause (global variable).vi" "pause core?"(FALSE ("pause core?")) -> ()
                  }
                }
                n167 = call "Enqueue--config_buttons.vi"("error in (no error)"=w244, "config_buttons"=config_buttons--enum."tour_running") -> ("error out"=w250:errorcluster)  [unwired: 9 in]
                n168 = property on="start" class="Bool"(error in=w250) -> (error out=w248:errorcluster, "BoolText.Text"=w247:string)  [unwired: 1 in, 1 out]
                n169 = case shown="\"START\"" w247 {
                  tunnel: [w255 w263 w280] -> w249
                  tunnel: w248 -> [w254 w270 w281]
                  tunnel: w243 -> [w256 w268 w278]
                  tunnel: [w256 w267 w278] -> w242
                  frame "RESUME" {
                    n170 = call "resume.vi"("error in"=w254) -> ("error out"=w255:errorcluster)  [unwired: 10 in]
                  }
                  frame "START" {
                    w264 = ""
                    w261 = u64 0 ("work.no. of complete tours")
                    # "The text log is created here. A new log is created every time user presses the \"START\" button. But not when user presses \"RESUME\"."
                    n171 = case shown="True" "Log reports to file?" {
                      tunnel: [_ w277] -> w272
                      tunnel: w270 -> [w274 w276]
                      tunnel: [w274 w275] -> w269
                      frame False {
                      }
                      frame True {
                        n172 = call "Create.vi"("error in (no error)"=w276) -> ("error out"=w275:errorcluster, "Log file path"=w277:path)  [unwired: 9 in]
                      }
                    }
                    n173 = Bundle By Name(cluster=w268, "complete_tours"=T4[] [], "no. of complete tours"=w261, "complete_tour currently displayed"=w261) -> (w267:T3)
                    n174 = Path To String(path=w272) -> (string=→"log file path":string)
                    n175 = local write "no. of complete tours"(w264) -> ()
                    n176 = local write "complete_tour"(w264) -> ()
                    n177 = call "Send command.vi"("error in (no error)"=w269, "command"="run_core") -> ("error out"=w258:errorcluster)  [unwired: 9 in]
                    n178 = call "start.vi"("error in"=w258) -> ("error out"=w257:errorcluster)  [unwired: 10 in]
                    n179 = To Variant(anything=T8 {"Completed tour paragraph"="", "tour number"=0} ("update_completed_tour_text_indicator arguments")) -> (Variant=w260:variant)
                    n180 = call "Enqueue MHL Queue-single.vi"("ErrorIn"=w257, "Data"=w260, "Command"="update_completed_tour_text_indicator" ("command")) -> ("ErrorOut"=w263:errorcluster)  [unwired: 8 in]
                  }
                  frame Default {
                    n181 = call "Raise assertion.vi"("error in (no error)"=w281, "Details (dflt=\"no details\")"="Boolean text not recognised") -> ("error out"=w280:errorcluster)  [unwired: 9 in]
                  }
                }
              }
              frame "button_press_pause" {
                n182 = call "pause.vi"("error in"=w282) -> ("error out"=w283:errorcluster)  [unwired: 10 in]
                n183 = global write "pause (global variable).vi" "pause core?"(TRUE ("pause core?")) -> ()
                n184 = call "Enqueue--config_buttons.vi"("error in (no error)"=w283, "config_buttons"=config_buttons--enum."tour_paused") -> ("error out"=w285:errorcluster)  [unwired: 9 in]
              }
              frame "button_press_stop" {
                n185 = call "pause.vi"("error in"=w290) -> ("error out"=w291:errorcluster)  [unwired: 10 in]
                n186 = call "Enqueue--config_buttons.vi"("error in (no error)"=w291, "config_buttons"=config_buttons--enum."tour_not_running") -> ("error out"=w292:errorcluster)  [unwired: 9 in]
                n187 = call "Set stop flag.vi"("error in (no error)"=w292) -> ("error out"=w289:errorcluster)  [unwired: 10 in]
                n188 = call "Close.vi"("error in (no error)"=w289) -> ("error out"=w288:errorcluster)  [unwired: 10 in]
              }
              frame "complete_tour_found" {
                # "append the newly completed tour to the list of completed tours"
                # "the first completed tour has order number 1 (counting starts from 1)"
                # "A new \"complete tour\" has been found."
                n189 = Variant To Data(error in=w312, type=T4 {"complete_tour"=[], "start square"="", "end square"="", "tour type"=enum."open", "start_time"=timestamp(0 s since 1904-01-01), "end_time"=timestamp(0 s since 1904-01-01), "duration (seconds)"=0.0, "duration (formatted string)"="", "no. of moves forward"=0, "no. of moves backward"=0, "total no. of moves since core started running"=0} ("completed_tour"), Variant=w311) -> (data=w303:T4, error out=w296:errorcluster)
                n190 = Unbundle By Name(w305) -> ("complete_tours"=w307:T4[])
                n191 = local read "Log reports to file?"() -> (w297:bool)
                n192 = Build Array (concatenate)(w307, w303) -> (w301:T4[])
                n193 = Array Size(array=w301) -> (size(s)=w302:i32)
                n194 = To Unsigned Quad Integer(1:w302) -> (0:w295:u64)
                "no. of completed tours" <- w295
                n195 = case shown="True" w297 {
                  tunnel: [w313 w319] -> w310
                  tunnel: w303 -> [_ w317]
                  tunnel: w295 -> [_ w316]
                  tunnel: w296 -> [w313 w315]
                  frame False {
                  }
                  frame True {
                    n196 = call "create completed tour report.vi"("report format"="Report format", "tour number"=w316, "completed_tour"=w317) -> ("completed tour (log paragraph)"=w318:string)
                    n197 = call "Write tour.vi"("error in (no error)"=w315, "Completed tour paragraph"=w318) -> ("error out"=w319:errorcluster)  [unwired: 9 in]
                  }
                }
                n198 = Bundle By Name(cluster=w305, "complete_tours"=w301, "no. of complete tours"=w295) -> (w306:T3)
                n199 = Not Equal?(x=u64 1, y=w295) -> (x != y?=w298:bool)
                n200 = local read "display_latest"() -> (w308:bool)
                n201 = case shown="True" w298 {
                  tunnel: ["1 tour found" ("format string") w323] -> w300
                  tunnel: w295 -> [_ w322]
                  frame False {
                  }
                  frame True {
                    n202 = call "Number (U64) to comma delimited string.vi"("Number"=w322) -> ("Comma delimited string"=w321:string)
                    n203 = Format Into String(format string="%s tours found", w321) -> (resulting string=w323:string)  [unwired: 2 in, 1 out]
                  }
                }
                "no. of complete tours" <- w300
                n204 = case shown="True" w308 {
                  tunnel: w310 -> [w325 w326]
                  tunnel: [w325 w327] -> w309
                  frame False {
                  }
                  frame True {
                    n205 = call "Enqueue MHL Queue-single.vi"("ErrorIn"=w326, "Command"="display_latest_completed_tour") -> ("ErrorOut"=w327:errorcluster)  [unwired: 9 in]
                  }
                }
              }
              frame "display_latest_completed_tour" {
                n206 = Unbundle By Name(w333) -> ("complete_tours"=w330:T4[])
                n207 = Empty Array?(array=w330) -> (empty?=w332:bool)
                n208 = Not(x=w332) -> (.not. x?=w331:bool)
                n209 = case shown="True" w331 {
                  tunnel: [w335 w339] -> w329
                  tunnel: w334 -> [w335 w342]
                  tunnel: w330 -> [_ w341]
                  frame False {
                  }
                  frame True {
                    # "Note: The tour number starts counting from 1 (not from 0)."
                    n210 = Array Size(array=w341) -> (size(s)=w340:i32)
                    n211 = To Unsigned Quad Integer(1:w340) -> (0:w336:u64)
                    n212 = To Variant(anything=w336) -> (Variant=w338:variant)
                    n213 = call "Enqueue MHL Queue-single.vi"("ErrorIn"=w342, "Data"=w338, "Command"="display_given_completed_tour") -> ("ErrorOut"=w339:errorcluster)  [unwired: 8 in]
                  }
                }
              }
              frame "display_given_completed_tour" {
                # "Decrement is necessary because\nThe tour number starts counting from 1.\nThe index in the \"completed_tours\" array starts counting from 0."
                n214 = Variant To Data(error in=w355, type=u64 0, Variant=w350) -> (data=w344:u64, error out=w351:errorcluster)
                n215 = Unbundle By Name(w354) -> ("complete_tours"=w353:T4[])
                n216 = Decrement(x=w344) -> (x-1=w347:u64)
                n217 = To Long Integer(number=w347) -> (32bit integer=w348:i32)
                n218 = Index Array(array=w353, index=w348) -> (element=w345:T4)
                n219 = local read "Report format"() -> (w343:T1)
                n220 = call "create completed tour report.vi"("report format"=w343, "tour number"=w344, "completed_tour"=w345) -> ("completed tour (log paragraph)"=w346:string)
                n221 = call "Enqueue--update_complete_tour_text_indicator.vi"("error in (no error)"=w351, "tour number"=w344, "Completed tour paragraph"=w346) -> ("error out"=w352:errorcluster)  [unwired: 8 in]
              }
              frame "update_completed_tour_text_indicator" {
                n222 = Variant To Data(error in=w368, type=T8 {"Completed tour paragraph"="", "tour number"=0} ("update_completed_tour_text_indicator arguments"), Variant=w367) -> (data=w365:T8, error out=w362:errorcluster)
                n223 = Unbundle By Name(w358) -> ("no. of complete tours"=w356:u64)
                n224 = Unbundle By Name(w365) -> ("Completed tour paragraph"=→"complete_tour":string, "tour number"=w357:u64)
                "complete_tour currently displayed" <- w357
                n225 = control-ref of="display_next"() -> (w360:refnum<vi>)
                n226 = control-ref of="display_previous"() -> (w359:refnum<vi>)
                n227 = call "config--display_next and display_previous.vi"("no. of completed_tours"=w356, "completed_tour currently displayed"=w357, "error in (no error)"=w362, "display_previous"=w359, "display_next"=w360) -> ("error out"=w361:errorcluster)  [unwired: 6 in]
                n228 = Bundle By Name(cluster=w358, "complete_tour currently displayed"=w357) -> (w363:T3)
              }
              frame "display_next_button_press" {
                n229 = Unbundle By Name(w374) -> ("no. of complete tours"=w370:u64, "complete_tour currently displayed"=w369:u64)
                n230 = Less?(x=w369, y=w370) -> (x < y?=w371:bool)
                n231 = case shown="True" w371 {
                  tunnel: w373 -> [w376 w382]
                  tunnel: [w377 w381] -> w372
                  tunnel: w369 -> [_ w380]
                  frame False {
                    n232 = call "Raise assertion.vi"("error in (no error)"=w376, "Details (dflt=\"no details\")"="The \"NEXT\" button was enabled when it shouldn't have been.") -> ("error out"=w377:errorcluster)  [unwired: 9 in]
                  }
                  frame True {
                    n233 = Increment(x=w380) -> (x+1=w378:u64)
                    n234 = To Variant(anything=w378) -> (Variant=w379:variant)
                    n235 = call "Enqueue MHL Queue-single.vi"("ErrorIn"=w382, "Data"=w379, "Command"="display_given_completed_tour") -> ("ErrorOut"=w381:errorcluster)  [unwired: 8 in]
                  }
                }
              }
              frame "display_previous_button_press" {
                n236 = Unbundle By Name(w389) -> ("complete_tour currently displayed"=w384:u64)
                n237 = Greater?(x=w384, y=u64 1) -> (0:w386:bool)
                n238 = case shown="True" w386 {
                  tunnel: w388 -> [w391 w398]
                  tunnel: [w392 w394] -> w387
                  tunnel: w384 -> [_ w397]
                  frame False {
                    n239 = call "Raise assertion.vi"("error in (no error)"=w391, "Details (dflt=\"no details\")"="The \"PREVIOUS\" button was enabled when it shouldn't have been.") -> ("error out"=w392:errorcluster)  [unwired: 9 in]
                  }
                  frame True {
                    # "Design\nTurn-off the \"Always display latest completed tour\" checkbox when user presses \"PREVIOUS\"."
                    n240 = Decrement(x=w397) -> (x-1=w395:u64)
                    n241 = To Variant(anything=w395) -> (Variant=w396:variant)
                    n242 = local write "display_latest"(FALSE ("display_latest")) -> ()
                    n243 = call "Enqueue MHL Queue-single.vi"("ErrorIn"=w398, "Data"=w396, "Command"="display_given_completed_tour") -> ("ErrorOut"=w394:errorcluster)  [unwired: 8 in]
                  }
                }
              }
            }
            n244 = call "Error Handler for MHL and EHL.vi"("ErrorIn"=w119) -> ("ErrorOut"=w117:errorcluster)  [unwired: 10 in]
            "MHL iteration" <- w114
          }
          n245 = while "core_loop" {
            shift-right: [w90] -> w49
            shift-left: w44 -> [w93]
            i -> [w94]
            stop <- w88 stop-if-true
            n246 = call "Receive command.vi"("error in (no error)"=w93) -> ("error out"=w92:errorcluster, "command"=w91:string)  [unwired: 8 in, 1 out]
            n247 = case shown="\"run_core\"" w91 {
              selector: w91 -> [w95 _ _ _ _]
              tunnel: w92 -> [w99 w102 w103 w104 w108]
              tunnel: [w98 w101 w103 w104 w108] -> w90
              tunnel: [_ _ _ _ TRUE] -> w87
              frame Default {
                n248 = Format Into String(format string="Unrecognised command in core_loop.\nCommand = %s" ("Details (dflt=\"no details\")"), w95) -> (resulting string=w96:string)  [unwired: 2 in, 1 out]
                n249 = call "Raise assertion.vi"("error in (no error)"=w99, "Details (dflt=\"no details\")"=w96) -> ("error out"=w98:errorcluster)  [unwired: 9 in]
              }
              frame "error" {
                n250 = call "error_handler_display_loops.vi"("error in (no error)"=w102, "Name of VI or Module"="run_core_loop") -> ("error out"=w101:errorcluster)  [unwired: 9 in]
              }
              frame "idle" {
                # "This case is expected to execute when there are no new messages. Do nothing."
              }
              frame "run_core" {
                w105 = T9 {"file"=enum."a", "rank"=enum."1"}  # starting_square
                w106 = u8 8  # chessboard_size
                n251 = call "main.vi"("chessboard_size"=w106, "starting_square"=w105) -> ()  [unwired: 1 in]
              }
              frame "exit_loop" {
              }
            }
            n252 = call "Read stop loops flag.vi"() -> ("Stop all loops?"=w89:bool)  [unwired: 10 in, 1 out]
            n253 = Or(x=w87, y=w89) -> (x .or. y?=w88:bool)
            "core loop" <- w94
          }
          n254 = while "display_loop_1" {
            shift-right: [w56] -> w48
            shift-left: w44 -> [w59]
            i -> [w60]
            stop <- w54 stop-if-true
            n255 = call "Receive command.vi"("error in (no error)"=w59) -> ("error out"=w58:errorcluster, "command"=w57:string)  [unwired: 8 in, 1 out]
            n256 = case shown="\"idle\"" w57 {
              selector: w57 -> [w61 _ _ _]
              tunnel: w58 -> [w65 w67 w84 w86]
              tunnel: [w64 w66 w72 w86] -> w56
              tunnel: [_ _ _ TRUE] -> w53
              frame Default {
                n257 = Format Into String(format string="Unrecognised command in display_loop.\nCommand = %s" ("Details (dflt=\"no details\")"), w61) -> (resulting string=w62:string)  [unwired: 2 in, 1 out]
                n258 = call "Raise assertion.vi"("error in (no error)"=w65, "Details (dflt=\"no details\")"=w62) -> ("error out"=w64:errorcluster)  [unwired: 9 in]
              }
              frame "error" {
                n259 = call "error_handler_display_loops.vi"("error in (no error)"=w67, "Name of VI or Module"="display_loop_2") -> ("error out"=w66:errorcluster)  [unwired: 9 in]
              }
              frame "idle" {
                n260 = call "read--tour_in_progress--tour.vi"() -> ("tour"=w81:T5[])
                n261 = call "draw current_tour on chessboard.vi"("current_tour"=w81) -> ("Chess board"=→"chessboard":bool[][])  [unwired: 10 in]
                n262 = call "convert--tour to string (in rows).vi"("tour"=w81) -> ("tour (string)"=→"The tour":string)
                n263 = call "read--total_no_of_moves.vi"() -> ("total no. of moves backward"=w78:u64, "total no. of moves forward"=w80:u64)  [unwired: 2 in]
                n264 = Add(x=w80, y=w78) -> (x+y=w75:u64)
                "total no. of moves" <- w75
                n265 = call "Number (U64) to comma delimited string.vi"("Number"=w80) -> ("Comma delimited string"=→"total no. of moves forward":string)
                n266 = call "Number (U64) to comma delimited string.vi"("Number"=w78) -> ("Comma delimited string"=→"total no. of moves backward":string)
                n267 = call "Number (U64) to comma delimited string.vi"("Number"=w75) -> ("Comma delimited string"=→"total no. of moves":string)
                n268 = call "get elapsed time.vi"("error in"=w84) -> ("error out"=w72:errorcluster, "time spent running (seconds)"=w71:dbl)  [unwired: 7 in, 2 out]
                n269 = local read "no. of completed tours"() -> (w69:u64)
                n270 = call "convert seconds to h min string.vi"("time duration (seconds)"=w71) -> ("running time string"=→"running time":string)
                n271 = call "get average move speed.vi"("time spent running (seconds)"=w71, "total no. of moves"=w75) -> ("avg. move speed (moves/second)"=→"avg. move speed":string)
                n272 = call "get average tour finding speed.vi"("time spent running (seconds)"=w71, "total no. of tours found"=w69) -> ("avg. tour finding speed (tours/second)"=→"avg. tour finding speed":string)
              }
              frame "exit_loop" {
              }
            }
            n273 = call "Read stop loops flag.vi"() -> ("Stop all loops?"=w55:bool)  [unwired: 10 in, 1 out]
            n274 = Or(x=w53, y=w55) -> (x .or. y?=w54:bool)
            "display loop 1" <- w60
          }
          n275 = while "display_loop_2" {
            shift-right: [w509] -> w46
            shift-left: w44 -> [w510]
            shift-right: [w506] -> _
            shift-left: w45 -> [w507]
            i -> [w511]
            stop <- w504 stop-if-true
            n276 = flat-sequence {
              tunnel: w510 -> [w517]
              tunnel: [w517] -> w508
              tunnel: w507 -> [w516]
              tunnel: [w515] -> w505
              tunnel: [w525] -> w509
              tunnel: w508 -> [w522]
              tunnel: [w524] -> w506
              tunnel: w505 -> [w524]
              tunnel: [w521] -> w504
              frame #0 {
                # "latest value"
                n277 = local read "total no. of moves"() -> (w515:u64)
                n278 = Less Or Equal?(x=w516, y=w515) -> (x <= y?=w514:bool)
                n279 = case shown="True" w514 {
                  tunnel: [_ w520] -> w513
                  tunnel: w516 -> [_ w519]
                  tunnel: w515 -> [_ w518]
                  frame False {
                    # "After a tour restart."
                  }
                  frame True {
                    # "normal case."
                    n280 = Subtract(x=w518, y=w519) -> (x-y=w520:u64)
                  }
                }
                n281 = call "Number (U64) to comma delimited string.vi"("Number"=w513) -> ("Comma delimited string"=→"no. of moves forward and backward in the last second":string)
              }
              frame #1 {
                n282 = call "Read stop loops flag.vi"("error in (no error)"=w522) -> ("error out"=w523:errorcluster, "Stop all loops?"=w521:bool)  [unwired: 9 in]
                n283 = case shown="False" w521 {
                  tunnel: w523 -> [w527 w528]
                  tunnel: [w526 w528] -> w525
                  frame False {
                    n284 = call "Wait 1000 ms.vi"("error in (no error)"=w527) -> ("error out"=w526:errorcluster)  [unwired: 10 in]
                  }
                  frame True {
                  }
                }
              }
            }
            "display loop 2" <- w511
          }
          n285 = Merge Errors(w52, w47, w49, w48, w46) -> (w51:errorcluster)
        }
        frame Error {
          # "Error during pre-loop initialisation. Skip loops. Exit VI."
        }
      }
      n286 = call "Close.vi"("error in (no error)"=w5) -> ("error out"=w4:errorcluster)  [unwired: 10 in]
      n287 = call "Destroy command queue.vi"("error in (no error)"=w4) -> ("error out"=w20:errorcluster)  [unwired: 10 in]
      n288 = call "Destroy command queue.vi"("error in (no error)"=w20) -> ("error out"=w29:errorcluster)  [unwired: 10 in]
    }
    frame Error {
    }
  }
  n289 = disable-structure shown="Disabled" {
    frame Disabled {
      (unwired) T3 {"complete_tours"=[], "no. of complete tours"=0, "complete_tour currently displayed"=0}  # Module Data
      # "Module data"
    }
    frame Enabled {
    }
  }
  n290 = disable-structure shown="Disabled" {
    frame Disabled {
      w531 = "<command>"  # Command
      w532 = string[] []  # Commands
      # "MHL queue"
      n291 = call "Enqueue MHL Queue-array.vi"("Commands"=w532) -> ()  [unwired: 10 in, 1 out]
      n292 = call "Enqueue MHL Queue-single.vi"("Command"=w531) -> ()  [unwired: 10 in, 1 out]
    }
    frame Enabled {
    }
  }
  n293 = disable-structure shown="Disabled" {
    frame Disabled {
      # "core loop queue"
      n294 = call "Create command queue.vi"() -> ()  [unwired: 11 in, 1 out]
      n295 = call "Destroy command queue.vi"() -> ()  [unwired: 11 in, 1 out]
      n296 = call "Receive command.vi"() -> ()  [unwired: 9 in, 3 out]
      n297 = call "Send command.vi"() -> ()  [unwired: 11 in, 1 out]
    }
    frame Enabled {
    }
  }
  n298 = disable-structure shown="Disabled" {
    frame Disabled {
      # "Commonly inspected VIs"
      n299 = call "main.vi"() -> ()  [unwired: 3 in]
    }
    frame Enabled {
    }
  }
  n300 = call "Quit LabVIEW if EXE.vi"("error in (no error)"=w2) -> ("error out"=→"error out":errorcluster)  [unwired: 10 in]
